vi "Example.vi"() -> ()   [LabVIEW 2024]
uses:
  Config Files Management/Config Files Management.lvlib
  Config Files Management/section data--cluster.ctl
panel:
  out "restitucion":T1
  out "despues borrado":T1
  out "antes borrado":T1
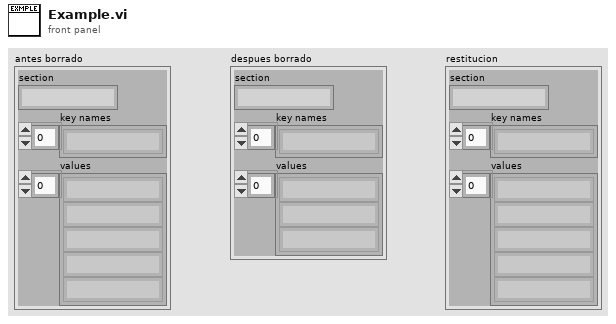
[diagram p1: front panel]
types:
  T1 = typedef "Config Files Management.lvlib/section data--cluster.ctl" = cluster{"section":string, "key names":string[], "values":string[]}
  T2 = typedef "NI_LVConfig.lvlib/Config Data RefNum.ctl" = refnum<k1>
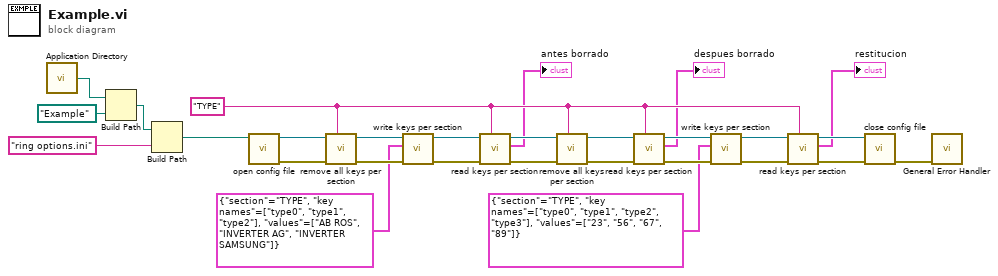
[diagram p0: block diagram]
diagram:
  w13 = "TYPE" ("section")
  n1 = call <vilib>:"Application Directory.vi"() -> ("Application Directory"=w5:path)
  n2 = Build Path(base path=w5, name or relative path=path "Example") -> (appended path=w2:path)
  n3 = Build Path(base path=w2, name or relative path="ring options.ini" ("file name")) -> (appended path=w1:path)
  n4 = call "open config file.vi"("configuration file path"=w1) -> ("error out"=w17:errorcluster, "Refnum out"=w16:T2)  [unwired: 8 in, 1 out]
  n5 = call "remove all keys per section.vi"("section"=w13, "error in (no error)"=w17, "Refnum in"=w16) -> ("error out"=w14:errorcluster, "Refnum out"=w15:T2)  [unwired: 7 in]
  n6 = call "write keys per section.vi"("error in (no error)"=w14, "section data"=T1 {"section"="TYPE", "key names"=["type0", "type1", "type2"], "values"=["AB ROS", "INVERTER AG", "INVERTER SAMSUNG"]}, "Refnum in"=w15) -> ("error out"=w12:errorcluster, "Refnum out"=w9:T2)  [unwired: 7 in]
  n7 = call "read keys per section.vi"("section"=w13, "error in (no error)"=w12, "Refnum in"=w9) -> ("error out"=w27:errorcluster, "section data"=→"antes borrado":T1, "Refnum out"=w26:T2)  [unwired: 6 in]
  n8 = call "remove all keys per section.vi"("section"=w13, "error in (no error)"=w27, "Refnum in"=w26) -> ("error out"=w25:errorcluster, "Refnum out"=w23:T2)  [unwired: 7 in]
  n9 = call "read keys per section.vi"("section"=w13, "error in (no error)"=w25, "Refnum in"=w23) -> ("error out"=w22:errorcluster, "section data"=→"despues borrado":T1, "Refnum out"=w21:T2)  [unwired: 6 in]
  n10 = call "write keys per section.vi"("error in (no error)"=w22, "section data"=T1 {"section"="TYPE", "key names"=["type0", "type1", "type2", "type3"], "values"=["23", "56", "67", "89"]}, "Refnum in"=w21) -> ("error out"=w20:errorcluster, "Refnum out"=w19:T2)  [unwired: 7 in]
  n11 = call "read keys per section.vi"("section"=w13, "error in (no error)"=w20, "Refnum in"=w19) -> ("error out"=w24:errorcluster, "section data"=→"restitucion":T1, "Refnum out"=w10:T2)  [unwired: 6 in]
  n12 = call "close config file.vi"("error in (no error)"=w24, "Refnum in"=w10) -> ("error out"=w28:errorcluster)  [unwired: 9 in]
  n13 = call <vilib>:"General Error Handler.vi"("error in (no error)"=w28) -> ()  [unwired: 10 in, 5 out]
